vi "ImageUpdateImage.vi"   [LabVIEW 2012, in "Image.lvclass"]
uses:
  classes/Image.lvclass
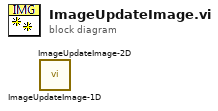
[diagram p0: block diagram]
diagram:
  n1 = call "ImageUpdateImage-1D.vi"() -> ()  [unwired: 9 in, 3 out]
  n2 = call "ImageUpdateImage-2D.vi"() -> ()  [unwired: 9 in, 3 out]
